vi "ComputeFisherMatrixFromLUT.vi"(9 "Show as dialog?":bool, 10 "MeasureConfig":T1={"Bead locations"=[{"X"=0, "Y"=0}], "ROI"=200, "Experiment base path"=path "", "Image output subdir"="images", "Output mode"=enum."None", "Traces output subdir"="traces", "QTrk Settings"={"Image width"=150, "Image height"=150, "Number of threads (CPU based)"=-1, "CUDA Device"=-2, "COM Background correction factor"=0.0, "ZLUT MinRadius"=8.0, "ZLUT Radial sample density"=5.0, "ZLUT Angular sample density"=2.0, "ZLUT ROI Coverage"=0.7, "QI Iterations"=1, "QI MinRadius"=2.0, "QI Radial sample density"=5.0, "QI Angular sample density"=2.0, "QI ROI Coverage"=0.7, "QI Angular Step \nIteration Factor"=0.8, "XCOR Profile Length"=1, "XCOR Profile Width"=128, "XCOR Iterations"=32, "Gaussian 2D Fit Iterations"=2, "Gaussian 2D Sigma (pixels)"=3.0, "Downsample"=0}, "Tracking Config"={"Number of steps"=0, "ZLUT stepsize (um)"=0.0, "Z correction factor"=0.0, "Start piezo Z (um)"=0.0, "Pixel size (nm)"=0.0, "2D Localization Type"=enum."Quadrant Interpolation", "Z Command (None)"=enum."ComputeZ", "Z Piezo scale"=FALSE}, "Experiment Name"="", "Program"={"Commands"=[], "Motor Axis accuracy conditions"={"Magnet Z"=0.0, "Magnet rotation"=0.0, "Camera"={"X"=0.0, "Y"=0.0}, "Piezo XY"={"X"=0.0, "Y"=0.0}, "Piezo Z"=0.0}, "Axis flags"={"Magnet Z"=FALSE, "Magnet rotation"=FALSE, "Camera"={"X"=FALSE, "Y"=FALSE}, "Piezo XY"={"X"=FALSE, "Y"=FALSE}, "Piezo Z"=FALSE}}, "ZLUT"=[], "Camera settings"={"Framerate (Hz)"=60, "Exposure time (us)"=5000, "Image size"={"Width"=1280, "Height"=1024}, "Number of buffers"=30}, "Experiment Script"="", "Max frames in memory"=2, "Save traces as binary"=FALSE, "Pixel Calibration Gain Image"="camera_calib_gain.bin", "Pixel Calibration Offset Image"="camera_calib_gain.bin", "Use pixel calibration images"=FALSE, "Internal camera settings"="", "Trace write interval"=100} {"QTrk Settings"."QI ROI Coverage" format="%_2g"; "QTrk Settings"."QI MinRadius" format="%.2f"; "QTrk Settings"."QI Angular sample density" format="%.3f"; "QTrk Settings"."QI Radial sample density" format="%.2f"; "QTrk Settings"."ZLUT Radial sample density" format="%.2f"; "QTrk Settings"."ZLUT MinRadius" format="%.2f"}, 11 "Bead index":i32) -> (3 "XY Graph":cluster{sgl[], dbl[]}[](graph))   [LabVIEW 2011]
uses:
  Typedefs/MeasureConfigType.ctl
  Typedefs/MeasureConfigOutputMode.ctl
  qtrk/QTrkLVBinding/QTrkSettings.ctl
  Typedefs/TrackingConfigType.ctl
  qtrk/QTrkLVBinding/QTrkLocalizationType.ctl
  qtrk/QTrkLVBinding/QTrkZCommandType.ctl
  ExperimentProgram/ExperimentProgramType.ctl
  ExperimentProgram/ExProgCommandType.ctl
  ExperimentProgram/ExProgCommandEnumType.ctl
  Motors/MotorAxisEnum.ctl
  Motors/MotorPosType.ctl
  Typedefs/XYf.ctl
  Motors/MotorPosFlagsType.ctl
  Camera/GenericCameraConfigType.ctl
panel:
  in  "Close dialog":bool
  out "Intensity Graph":sgl[][](graph)
  # "(used for commands with string parameters)"
  # "-2: Use all devices\n-1: Use best device"
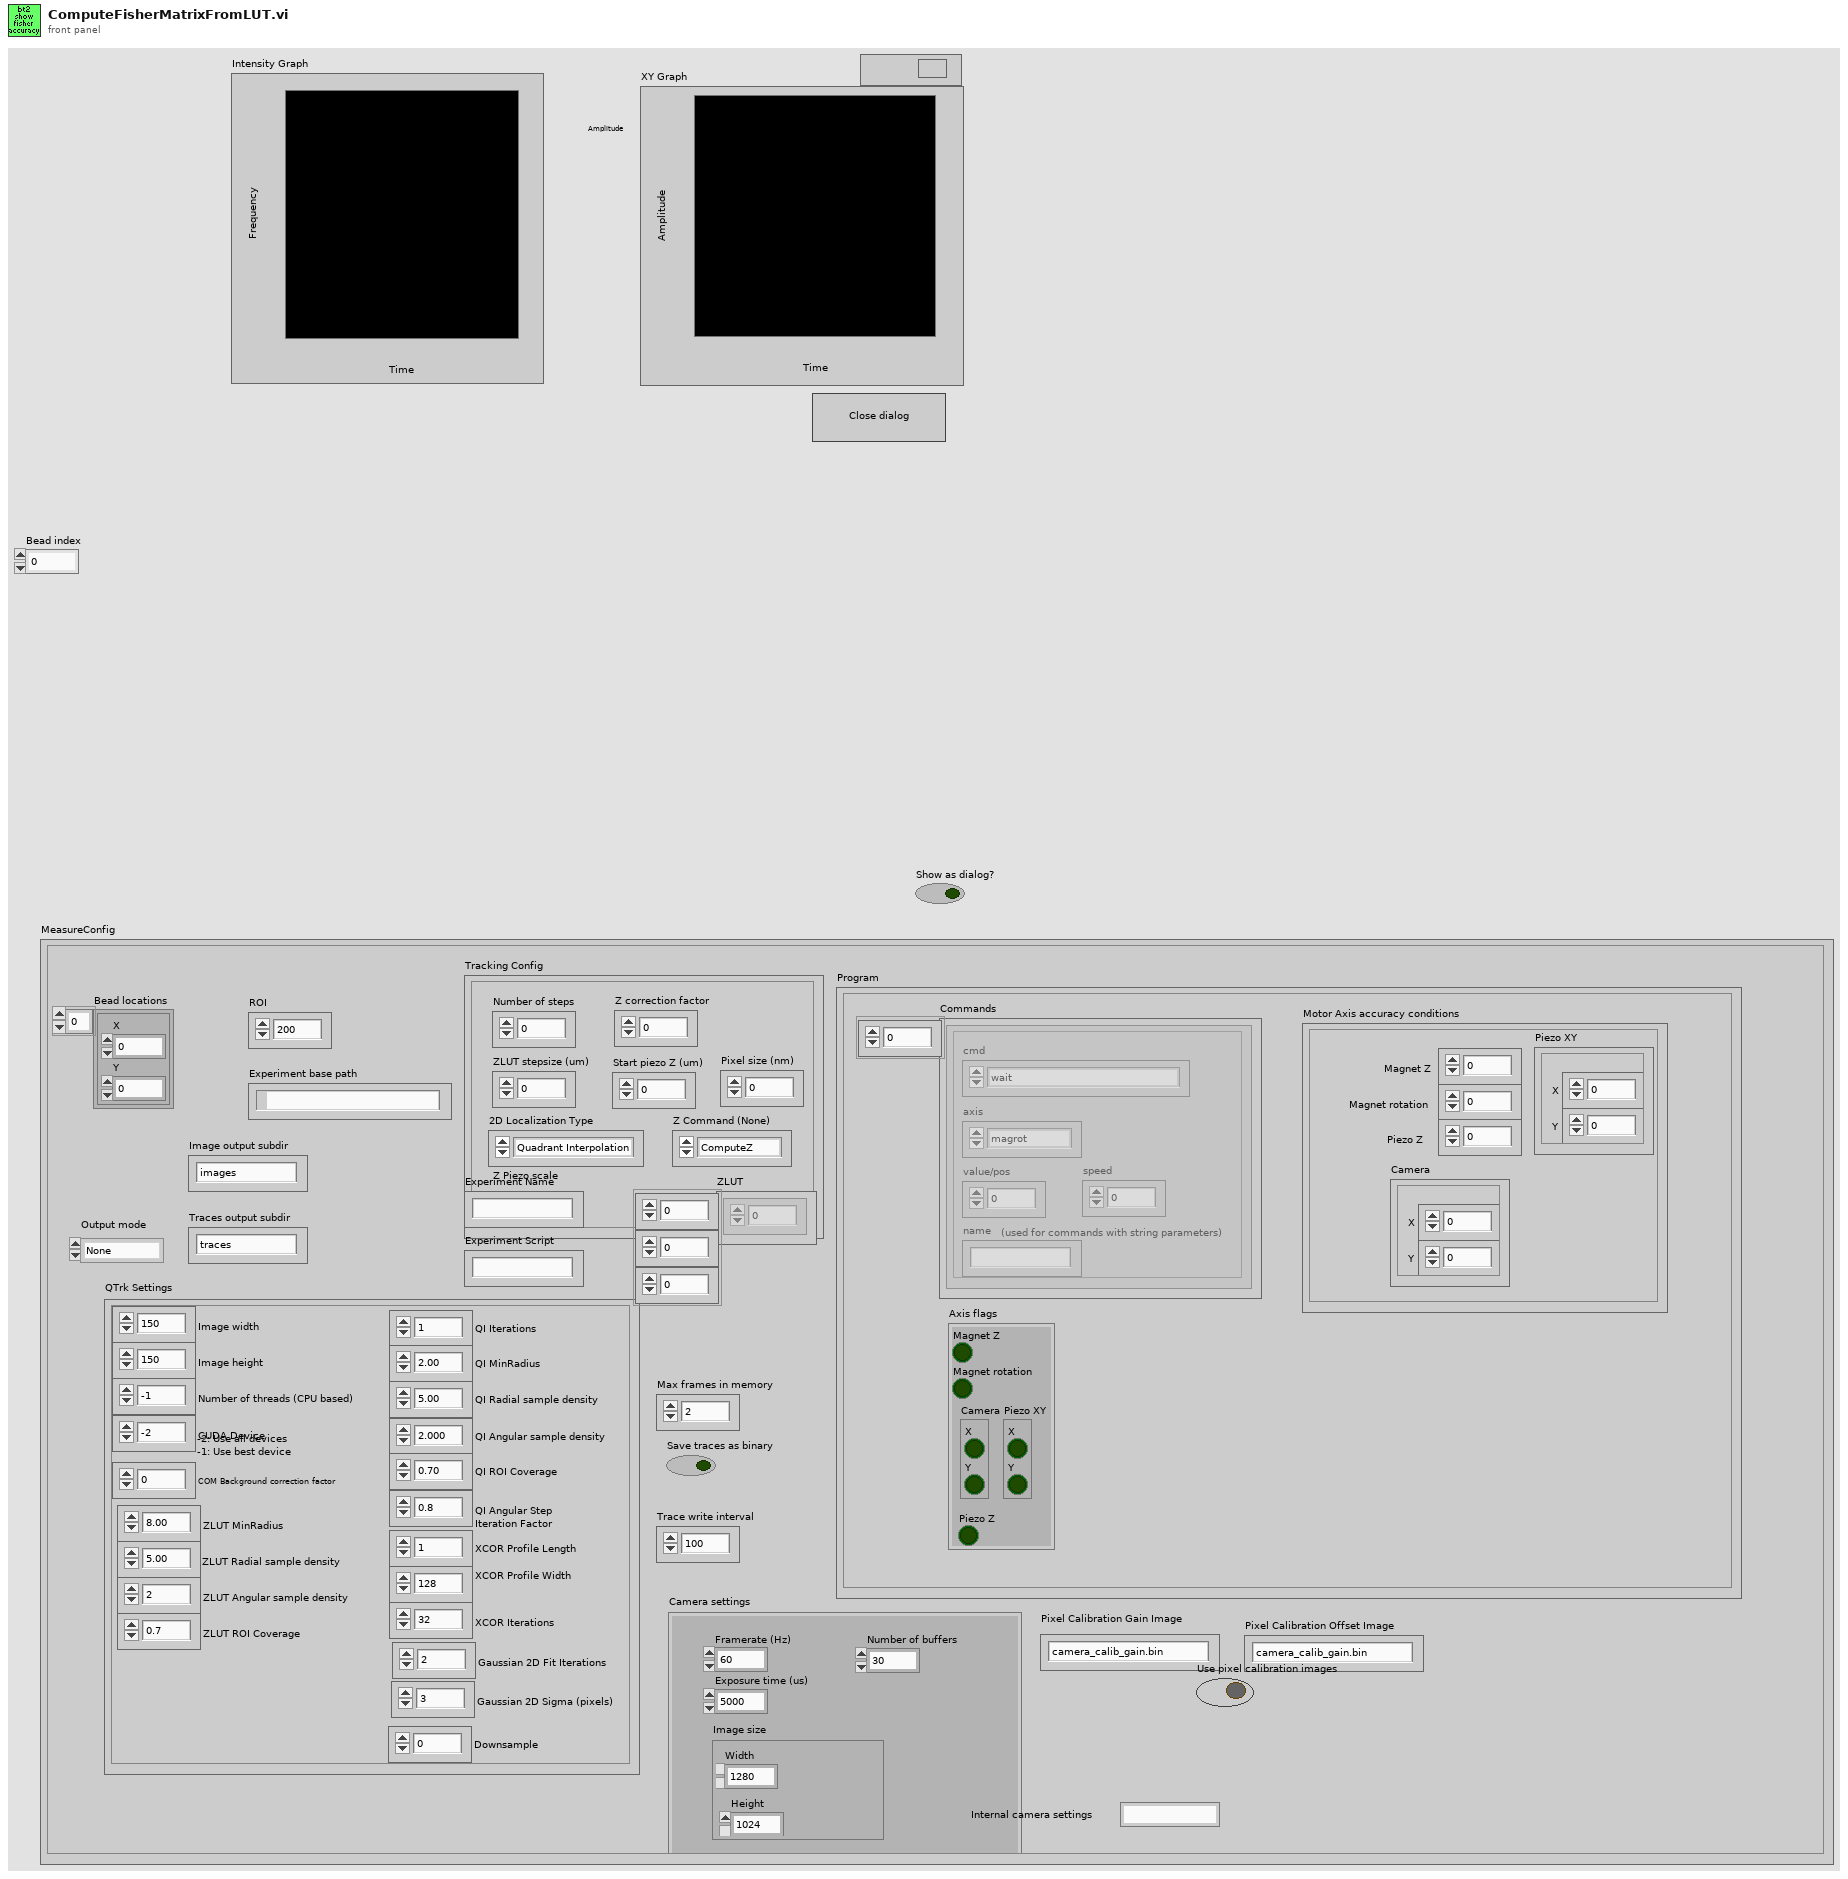
[diagram p1: front panel]
types:
  T1 = typedef "MeasureConfigType.ctl" = cluster{"Bead locations":cluster{"X":i32, "Y":i32}[], "ROI":i32, "Experiment base path":path, "Image output subdir":string, "Output mode":T2, "Traces output subdir":string, "QTrk Settings":T3, "Tracking Config":T4, "Experiment Name":string, "Program":T7, "ZLUT":sgl[][][], "Camera settings":T14, "Experiment Script":string, "Max frames in memory":i32, "Save traces as binary":bool, "Pixel Calibration Gain Image":string, "Pixel Calibration Offset Image":string, "Use pixel calibration images":bool, "Internal camera settings":string, "Trace write interval":i32}
  T2 = typedef "MeasureConfigOutputMode.ctl" = enum16{"None", "Track", "SaveImages"}
  T3 = typedef "QTrkSettings.ctl" = cluster{"Image width":i32, "Image height":i32, "Number of threads (CPU based)":i32, "CUDA Device":i32, "COM Background correction factor":sgl, "ZLUT MinRadius":sgl, "ZLUT Radial sample density":sgl, "ZLUT Angular sample density":sgl, "ZLUT ROI Coverage":sgl, "QI Iterations":i32, "QI MinRadius":sgl, "QI Radial sample density":sgl, "QI Angular sample density":sgl, "QI ROI Coverage":sgl, "QI Angular Step \nIteration Factor":sgl, "XCOR Profile Length":i32, "XCOR Profile Width":i32, "XCOR Iterations":i32, "Gaussian 2D Fit Iterations":i32, "Gaussian 2D Sigma (pixels)":sgl, "Downsample":i32}
  T4 = typedef "TrackingConfigType.ctl" = cluster{"Number of steps":i32, "ZLUT stepsize (um)":sgl, "Z correction factor":sgl, "Start piezo Z (um)":sgl, "Pixel size (nm)":sgl, "2D Localization Type":T5, "Z Command (None)":T6, "Z Piezo scale":bool}
  T5 = typedef "QTrkLocalizationType.ctl" = enum16{"Center-of-Mass", "1D Cross-Correlation", "Quadrant Interpolation", "Gaussian 2D MLE", "QI + ZLUTAlign", "ZLUTAlign", "QI + FourierLUT"}
  T6 = typedef "QTrkZCommandType.ctl" = enum16{"Nothing", "ComputeZ", "BuildRadialZLUT", "BuildImageZLUT", "RadialZLUT+ImageZLUT"}
  T7 = typedef "ExperimentProgramType.ctl" = cluster{"Commands":T8[], "Motor Axis accuracy conditions":T11, "Axis flags":T13}
  T8 = typedef "ExProgCommandType.ctl" = cluster{"cmd":T9, "axis":T10, "value/pos":dbl, "speed":dbl, "name":string}
  T9 = typedef "ExProgCommandEnumType.ctl" = enum16{"wait", "move", "acquire", "idle", "rmove", "when", "section", "stop"}
  T10 = typedef "MotorAxisEnum.ctl" = enum16{"no axis", "magrot", "magpos", "px", "py", "pz", "camx", "camy"}
  T11 = typedef "MotorPosType.ctl" = cluster{"Magnet Z":dbl, "Magnet rotation":dbl, "Camera":T12, "Piezo XY":T12, "Piezo Z":dbl}
  T12 = typedef "XYf.ctl" = cluster{"X":sgl, "Y":sgl}
  T13 = typedef "MotorPosFlagsType.ctl" = cluster{"Magnet Z":bool, "Magnet rotation":bool, "Camera":cluster{"X":bool, "Y":bool}, "Piezo XY":cluster{"X":bool, "Y":bool}, "Piezo Z":bool}
  T14 = typedef "GenericCameraConfigType.ctl" = cluster{"Framerate (Hz)":i32, "Exposure time (us)":i32, "Image size":cluster{"Width":i32, "Height":i32}, "Number of buffers":i32}
  T15 = typedef "XYZf.ctl" = cluster{"X":sgl, "Y":sgl, "Z":sgl}
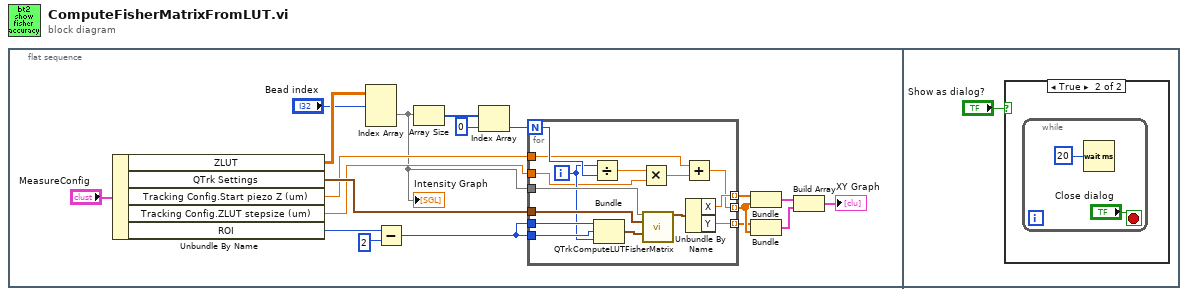
[diagram p0: block diagram]
diagram:
  n1 = flat-sequence {
    frame #0 {
      n2 = Unbundle By Name("MeasureConfig") -> ("ZLUT"=w15:sgl[][][], "QTrk Settings"=w13:T3, "Tracking Config.Start piezo Z (um)"=w9:sgl, "Tracking Config.ZLUT stepsize (um)"=w8:sgl, "ROI"=w12:i32)
      n3 = Index Array(array=w15, index (dim 0)="Bead index") -> (element=w1:sgl[][])  [unwired: 2 in]
      "Intensity Graph" <- w1
      n4 = Subtract(x=w12, y=2) -> (x-y=w10:i32)
      n5 = Array Size(array=w1) -> (size(s)=w19:i32[])
      n6 = Index Array(array=w19, index=0) -> (element=w17:i32)
      n7 = for {
        N: w17 -> [w33]
        tunnel: w1 -> [w34]
        tunnel: w13 -> [w31]
        tunnel: [w30] -> w6 mode=indexing
        tunnel: [w29] -> w5 mode=indexing
        tunnel: w10 -> [w27]
        tunnel: w10 -> [w26]
        tunnel: w9 -> [w24]
        tunnel: w8 -> [w22]
        tunnel: [w20] -> w7 mode=indexing
        i -> [w25]
        n8 = Divide(x=w25, y=w33) -> (x/y=w23:dbl)
        n9 = Bundle(w27, w26, w25) -> (w28:cluster{i32, i32, i32})  [unwired: 1 in]
        n10 = Multiply(x=w23, y=w22) -> (x*y=w21:dbl)
        n11 = call "QTrkComputeLUTFisherMatrix.vi"("LUT"=w34, "QTrk Settings"=w31, "XYZ"=w28) -> ("XYZ Variance"=w32:T15)  [unwired: 10 in, 2 out]
        n12 = Add(x=w24, y=w21) -> (x+y=w20:dbl)
        n13 = Unbundle By Name(w32) -> ("X"=w30:sgl, "Y"=w29:sgl)
      }
      n14 = Bundle(w6, w7) -> (w4:cluster{sgl[], dbl[]})  [unwired: 1 in]
      n15 = Bundle(w5, w7) -> (w3:cluster{sgl[], dbl[]})  [unwired: 1 in]
      n16 = Build Array(w4, w3) -> (→"XY Graph":cluster{sgl[], dbl[]}[])
    }
    frame #1 {
      n17 = case shown="True" "Show as dialog?" {
        frame False {
        }
        frame True {
          n18 = while {
            stop <- "Close dialog" stop-if-true
            n19 = Wait (ms)(milliseconds to wait=u32 20) -> ()  [unwired: 1 out]
          }
        }
      }
    }
  }
